vi "Disabled.vi"(7 "Robot Mode":T2, 10 "Match Info":T1={"Autonomous Elapsed Seconds"=0.0, "TeleOp Elapsed Seconds"=0.0, "Disabled Elapsed Seconds"=0.0, "Visited Autonomous"=FALSE, "Visited TeleOp"=FALSE, "Visited Disabled"=FALSE, "Autonomous Settings"={"Autonomous Style"=enum."Independent", "VI Refnum"=refnum}}, 11 "Call Context":T3) -> ()   [LabVIEW 2012]
doc: "This VI is called each time a disabled packet is received from the DS. It is often used to prepare for the next robot mode, to calibrate sensors, etc."
uses:
  <vilib>/Rock Robotics/WPI/DriverStation/WPI_DriverStationDerivedRobotMode.ctl
  <vilib>/Rock Robotics/WPI/DriverStation/WPI_DriverStationRobotMode2.ctl
  <vilib>/Rock Robotics/WPI/DriverStation/WPI_DriverStationMatch Info.ctl
  <vilib>/Rock Robotics/WPI/DriverStation/DriverStationLCD/WPI_DriverStationLCDLCDLine.ctl
  <vilib>/Rock Robotics/WPI/Joystick/WPI_JoystickGetSetRefNum.vi
  <vilib>/Utility/file.llb/Read From Spreadsheet File (string).vi
panel:
  out "handles the error":errorcluster
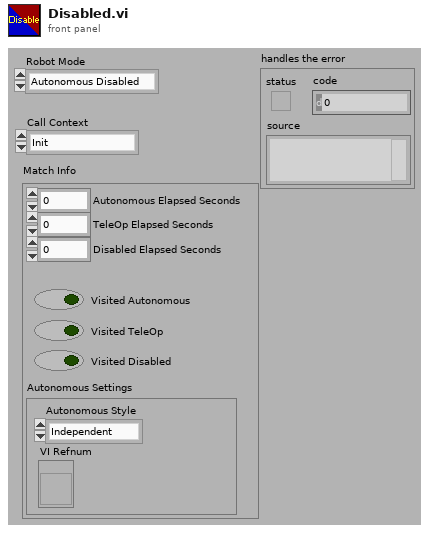
[diagram p1: front panel]
types:
  T1 = typedef "WPI_DriverStationMatch Info.ctl" = cluster{"Autonomous Elapsed Seconds":dbl, "TeleOp Elapsed Seconds":dbl, "Disabled Elapsed Seconds":dbl, "Visited Autonomous":bool, "Visited TeleOp":bool, "Visited Disabled":bool, "Autonomous Settings":cluster{"Autonomous Style":enum16{"Iterative", "Independent"}, "VI Refnum":refnum<vi>}}
  T2 = typedef "WPI_DriverStationRobotMode2.ctl" = enum16{"Autonomous Disabled", "Autonomous Enabled", "Teleop Disabled", "Teleop Enabled", "Timeout", "Finish", "Test Disabled", "Test Enabled"}
  T3 = typedef "WPI_DriverStationDerivedRobotMode.ctl" = enum16{"Init", "Execute", "Stop"}
  T4 = typedef "WPI_DriverStationLCDLCDLine.ctl" = enum16{"Main - Line 1", "User - Line 2", "User - Line 3", "User - Line 4", "User - Line 5", "User - Line 6"}
  T5 = typedef "WPI_JoystickDevRef.ctl" = cluster{"Device":T6}
  T6 = typedef "WPI_JoystickDeviceEnum.ctl" = enum16{"USB 1", "USB 2", "USB 3", "USB 4", "Kinect 1", "Kinect 2"}
  T7 = typedef "WPI_JoystickButtonState.ctl" = cluster{"Button 1":bool, "Button 2":bool, "Button 3":bool, "Button 4":bool, "Button 5":bool, "Button 6":bool, "Button 7":bool, "Button 8":bool, "Button 9":bool, "Button 10":bool, "Button 11":bool, "Button 12":bool}
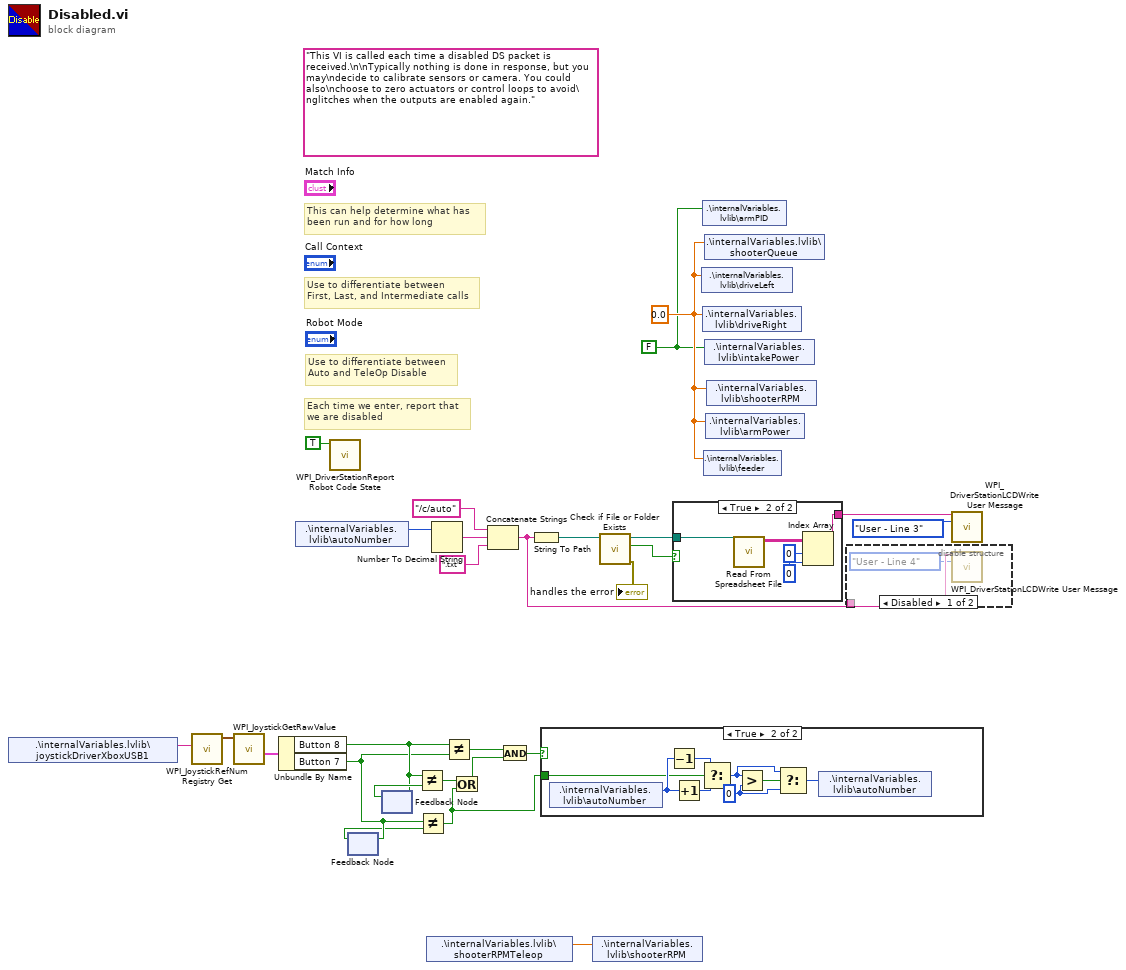
[diagram p0: block diagram]
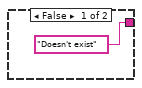
[diagram p3: hidden frame]
diagram:
  w1 = FALSE ("intakePower")
  w5 = 0.0 ("driveLeft")
  (unwired) "This VI is called each time a disabled DS packet is received.\n\nTypically nothing is done in response, but you may\ndecide to calibrate sensors or camera. You could also\nchoose to zero actuators or control loops to avoid\nglitches when the outputs are enabled again."
  # "Each time we enter, report that\nwe are disabled"
  # "Use to differentiate between\nFirst, Last, and Intermediate calls"
  # "This can help determine what has\nbeen run and for how long"
  # "Use to differentiate between\nAuto and TeleOp Disable"
  n1 = shared-variable ".\\internalVariables.lvlib\\joystickDriverXboxUSB1"() -> (w3:string)  [unwired: 1 in, 1 out]
  n2 = call <vilib>:"WPI_JoystickRefNum Registry Get.vi"("refnum name"=w3) -> ("JoystickDevRef"=w20:T5)  [unwired: 9 in, 1 out]
  n3 = call <vilib>:"WPI_JoystickGetRawValue.vi"("JoystickDevRef"=w20) -> ("Buttons"=w19:T7)  [unwired: 8 in, 2 out]
  n4 = Unbundle By Name(w19) -> ("Button 8"=w15:bool, "Button 7"=w14:bool)
  n5 = shared-variable ".\\internalVariables.lvlib\\autoNumber"() -> (w22:i16)  [unwired: 1 in, 1 out]
  n6 = call <vilib>:"WPI_DriverStationReport Robot Code State.vi"("Disabled"=TRUE ("Autonomous")) -> ()  [unwired: 10 in, 1 out]
  n7 = feedback #1() -> (w13:bool)  [unwired: 1 in]
  n8 = feedback-in #1(w14) -> ()
  n9 = feedback-in #2(w15) -> ()
  n10 = feedback #2() -> (w16:bool)  [unwired: 1 in]
  n11 = Not Equal?(x=w15, y=w16) -> (x != y?=w12:bool)
  n12 = Not Equal?(x=w14, y=w13) -> (x != y?=w10:bool)
  n13 = shared-variable ".\\internalVariables.lvlib\\shooterRPMTeleop"() -> (w2:dbl)  [unwired: 1 in, 1 out]
  n14 = Number To Decimal String(number=w22) -> (decimal integer string=w24:string)  [unwired: 1 in]
  n15 = Not Equal?(x=w15, y=w14) -> (x != y?=w17:bool)
  n16 = Or(x=w12, y=w10) -> (x .or. y?=w11:bool)
  n17 = Concatenate Strings("/c/auto", w24, ".txt" ("string")) -> (w7:string)
  n18 = And(x=w17, y=w11) -> (x .and. y?=w18:bool)
  n19 = String To Path(string=w7) -> (path=w6:path)
  n20 = case shown="True" w18 {
    tunnel: w10 -> [_ w31]
    frame False {
    }
    frame True {
      w29 = i16 0 ("y")
      n21 = shared-variable ".\\internalVariables.lvlib\\autoNumber"() -> (w33:i16)  [unwired: 1 in, 1 out]
      n22 = Decrement(x=w33) -> (x-1=w32:i16)
      n23 = Increment(x=w33) -> (x+1=w34:i16)
      n24 = Select(t=w32, s=w31, f=w34) -> (s? t:f=w28:i16)
      n25 = Greater?(x=w28, y=w29) -> (0:w30:bool)
      n26 = Select(t=w28, s=w30, f=w29) -> (s? t:f=w27:i16)
      n27 = shared-variable ".\\internalVariables.lvlib\\autoNumber"(w27) -> ()  [unwired: 1 in, 1 out]
    }
  }
  n28 = shared-variable ".\\internalVariables.lvlib\\shooterRPM"(w2) -> ()  [unwired: 1 in, 1 out]
  n29 = call <vilib>:"Check if File or Folder Exists.vi"("path"=w6) -> ("error out"=→"handles the error":errorcluster, "file or folder exists?"=w9:bool)  [unwired: 8 in, 1 out]
  n30 = case shown="True" w9 {
    tunnel: ["Doesn't exist" ("String") w37] -> w8
    tunnel: w6 -> [_ w36]
    frame False {
    }
    frame True {
      n31 = call-poly <vilib>:"Read From Spreadsheet File.vi"("file path (dialog if empty)"=w36) -> ("all rows"=w38:string[][])  [unwired: 6 in, 4 out]
      n32 = Index Array(array=w38, index (row)=0, index (col)=0 ("disabled index (col)")) -> (element=w37:string)
    }
  }
  n33 = shared-variable ".\\internalVariables.lvlib\\driveLeft"(w5) -> ()  [unwired: 1 in, 1 out]
  n34 = shared-variable ".\\internalVariables.lvlib\\armPID"(w1) -> ()  [unwired: 1 in, 1 out]
  n35 = shared-variable ".\\internalVariables.lvlib\\driveRight"(w5) -> ()  [unwired: 1 in, 1 out]
  n36 = shared-variable ".\\internalVariables.lvlib\\feeder"(w5) -> ()  [unwired: 1 in, 1 out]
  n37 = shared-variable ".\\internalVariables.lvlib\\shooterQueue"(w5) -> ()  [unwired: 1 in, 1 out]
  n38 = shared-variable ".\\internalVariables.lvlib\\intakePower"(w1) -> ()  [unwired: 1 in, 1 out]
  n39 = shared-variable ".\\internalVariables.lvlib\\armPower"(w5) -> ()  [unwired: 1 in, 1 out]
  n40 = shared-variable ".\\internalVariables.lvlib\\shooterRPM"(w5) -> ()  [unwired: 1 in, 1 out]
  n41 = disable-structure shown="Disabled" {
    disable-tunnel: w7 -> [w42 _]
    frame Disabled {
      n42 = call <vilib>:"WPI_DriverStationLCDWrite User Message.vi"("line text"=w42, "line"=WPI_DriverStationLCDLCDLine."User - Line 4") -> ()  [unwired: 13 in, 1 out]
    }
    frame Enabled {
    }
  }
  n43 = call <vilib>:"WPI_DriverStationLCDWrite User Message.vi"("line text"=w8, "line"=WPI_DriverStationLCDLCDLine."User - Line 3") -> ()  [unwired: 13 in, 1 out]
